vi "TDT-Get Tosca Markers.vi"(0 "Data":T1={"TTankX"=refnum, "TDevAccX"=refnum, "LastTime"=0.0, "error"={"status"=FALSE, "code"=0, "source"=""}, "Block Name"="", "Circuit Tag"="", "Tank Name"="", "NumTicks"=0, "LastTick"=0.0, "Idle?"=FALSE, "Wait (ms)"=1000, "LastArtf"=0.0, "LastTosc"=0.0}, 5 "T2":dbl, 7 "Max Read":i32=1000, 11 "error in (no error)":errorcluster) -> (4 "Got em' all":bool, 8 "Tosca markers":dbl[][](array[numeric]), 15 "error out":errorcluster)   [LabVIEW 2015]
uses:
  TDT Interface Data.ctl
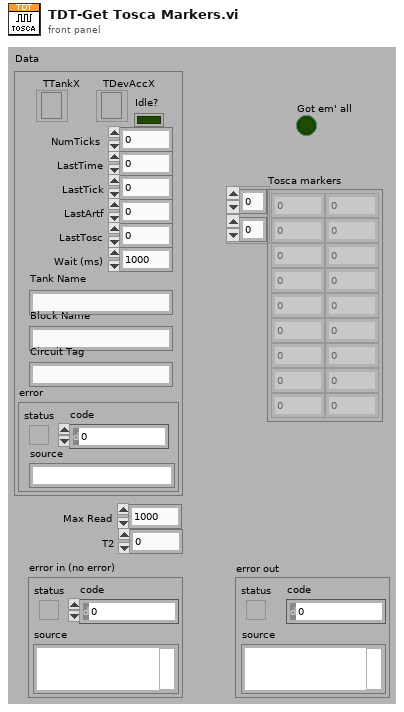
[diagram p1: front panel]
types:
  T1 = typedef "TDT Interface Data.ctl" = cluster{"TTankX":refnum<k7>, "TDevAccX":refnum<k7>, "LastTime":dbl, "error":errorcluster, "Block Name":string, "Circuit Tag":string, "Tank Name":string, "NumTicks":i32, "LastTick":dbl, "Idle?":bool, "Wait (ms)":u32, "LastArtf":dbl, "LastTosc":dbl}
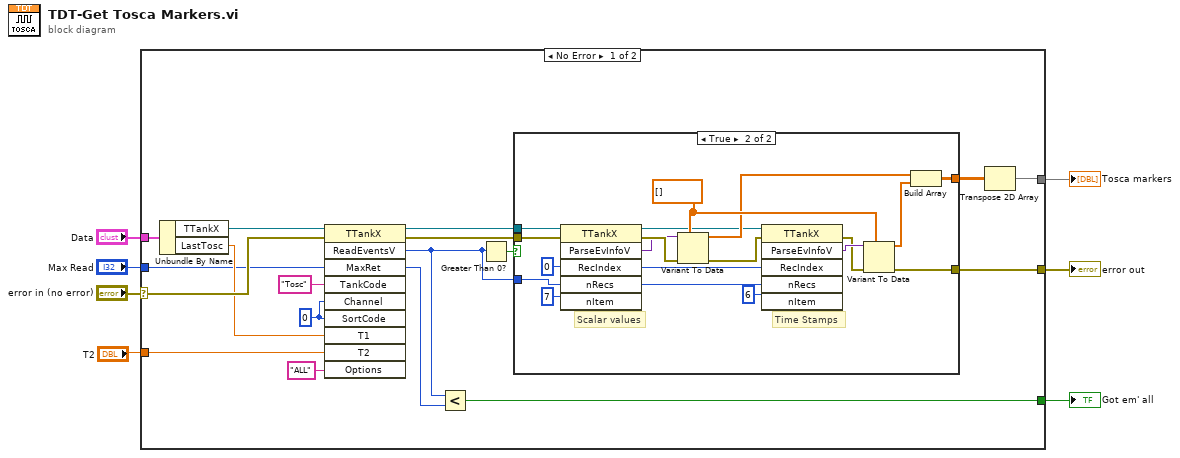
[diagram p0: block diagram]
diagram:
  n1 = case shown="No Error" "error in (no error)" {
    selector: "error in (no error)" -> [w23 w46]
    tunnel: "Data" -> [w25 _]
    tunnel: [w8 w46] -> w5
    tunnel: [w21 _] -> w4
    tunnel: "T2" -> [w13 _]
    tunnel: [w12 _] -> w2
    tunnel: "Max Read" -> [w10 _]
    frame No Error {
      w18 = 0 ("Channel")
      n2 = Unbundle By Name(w25) -> ("TTankX"=w24:refnum<k7>, "LastTosc"=w22:dbl)
      n3 = invoke class="TTankX" method="ReadEventsV"(reference=w24, error in=w23, "MaxRet"=w10, "TankCode"="Tosc", "Channel"=w18, "SortCode"=w18, "T1"=w22, "T2"=w13, "Options"="ALL") -> (reference out=w11:refnum<k7>, error out=w15:errorcluster, "ReadEventsV"=w14:i32, "MaxRet"=w16:i32)  [unwired: 1 in, 6 out]
      n4 = Less?(x=w14, y=w16) -> (x < y?=w12:bool)
      n5 = Greater Than 0?(x=w14) -> (x > 0?=w9:bool)
      n6 = case shown="True" w9 {
        tunnel: w11 -> [_ w45]
        tunnel: w15 -> [w26 w44]
        tunnel: w14 -> [_ w42]
        tunnel: [_ w32] -> w20
        tunnel: [w26 w37] -> w8
        frame False {
        }
        frame True {
          w33 = dbl[] []
          # "Time Stamps"
          # "Scalar values"
          n7 = invoke class="TTankX" method="ParseEvInfoV"(reference=w45, error in=w44, "RecIndex"=0, "nRecs"=w42, "nItem"=7) -> (reference out=w30:refnum<k7>, error out=w40:errorcluster, "ParseEvInfoV"=w34:variant, "RecIndex"=w28:i32, "nRecs"=w27:i32)  [unwired: 1 in, 1 out]
          n8 = Variant To Data(error in=w40, type=w33, Variant=w34) -> (data=w31:dbl[], error out=w29:errorcluster)
          n9 = invoke class="TTankX" method="ParseEvInfoV"(reference=w30, error in=w29, "RecIndex"=w28, "nRecs"=w27, "nItem"=6) -> (error out=w36:errorcluster, "ParseEvInfoV"=w38:variant)  [unwired: 1 in, 4 out]
          n10 = Variant To Data(error in=w36, type=w33, Variant=w38) -> (data=w35:dbl[], error out=w37:errorcluster)
          n11 = Build Array(w31, w35) -> (w32:dbl[][])
        }
      }
      n12 = Transpose 2D Array(2D array=w20) -> (transposed array=w21:dbl[][])
    }
    frame Error {
    }
  }
  "Tosca markers" <- w4
  "error out" <- w5
  "Got em' all" <- w2
